vi "Find Web Methods.vi"(11 "Project":path) -> (2 "Web Methods":path[](array[path]))   [LabVIEW 2014]
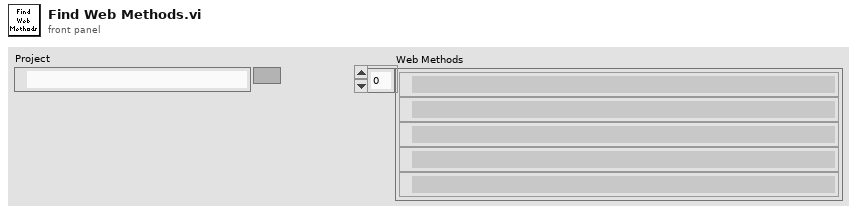
[diagram p1: front panel]
types:
  T1 = typedef "NI_FileType.lvlib/LVFileType.ctl" = enum32{"Invalid file", "Unknown type", "Instrument", "Control", "Polymorphic VI", "Project", "Library", "LVClass", "XControl", "XNode", "Shared library", ".NET assembly", "ActiveX interface", "CIN", "Run-time menu", "Palette menu", "Help file", "LLB", "XNode Edit Dependency", "Class Private Data Control", "Statechart", "MathScript .m file", "Ladder Diagram", "LVLibp", "XNode Build Dependency"}
  T2 = cluster{"path":path, "delimited name":string, "type":T1, "iState":u32, "iStyle":u16, "wStyle":u16, "buttons":u16, "viflags":u32, "viflags2":u32, "links":u32[]}[]
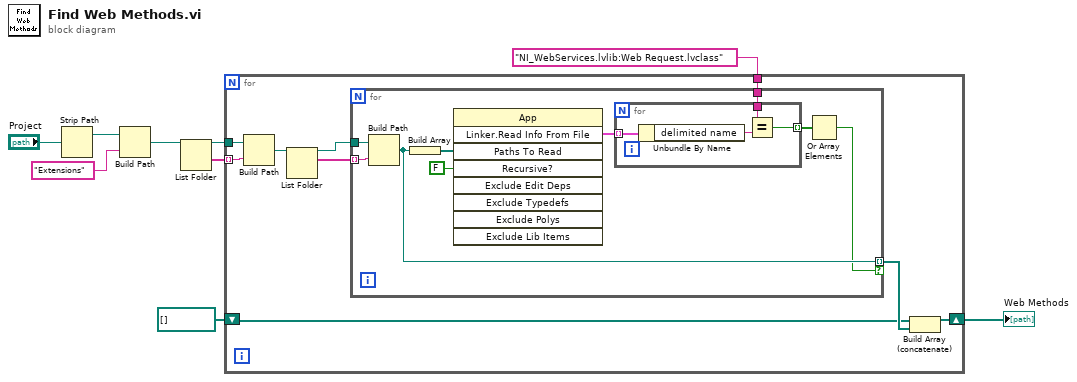
[diagram p0: block diagram]
diagram:
  n1 = Strip Path(path="Project") -> (stripped path=w5:path)  [unwired: 1 out]
  n2 = Build Path(base path=w5, name or relative path="Extensions") -> (appended path=w7:path)
  n3 = List Folder(path=w7) -> (path out=w9:path, folder names=w8:string[])  [unwired: 3 in, 2 out]
  n4 = for {
    tunnel: w8 -> [w17] mode=indexing
    tunnel: w9 -> [w18]
    tunnel: "NI_WebServices.lvlib:Web Request.lvclass" ("class name") -> [w13]
    shift-right: [w12] -> w3
    shift-left: path[] [] -> [w10]
    n5 = Build Path(base path=w18, name or relative path=w17) -> (appended path=w16:path)
    n6 = List Folder(path=w16) -> (path out=w14:path, filenames=w15:string[])  [unwired: 3 in, 2 out]
    n7 = for {
      tunnel: w15 -> [w27] mode=indexing
      tunnel: w14 -> [w26]
      tunnel: w13 -> [w23]
      tunnel: [w21] -> w11 mode=indexing if=w20
      n8 = Build Path(base path=w26, name or relative path=w27) -> (appended path=w21:path)
      n9 = Build Array(w21) -> (w25:path[])
      n10 = invoke class="App" method="Linker.Read Info From File"("Paths To Read"=w25, "Recursive?"=FALSE) -> ("Linker.Read Info From File"=w24:T2)  [unwired: 7 in, 8 out]
      n11 = for {
        tunnel: w24 -> [w31] mode=indexing
        tunnel: w23 -> [w29]
        tunnel: [w28] -> w22 mode=indexing
        n12 = Unbundle By Name(w31) -> ("delimited name"=w30:string)
        n13 = Equal?(x=w29, y=w30) -> (x = y?=w28:bool)
      }
      n14 = Or Array Elements(Boolean array=w22) -> (logical OR=w20:bool)
    }
    n15 = Build Array (concatenate)(w10, w11) -> (w12:path[])
  }
  "Web Methods" <- w3
